vi "Process-images.vi"(8 "error in":errorcluster, 10 "UI ref. in":refnum<data-value>, 11 "Data ref. in":refnum<data-value>) -> (0 "error IO":errorcluster, 2 "UI ref.":refnum<data-value>, 3 "Data ref.":refnum<data-value>)   [LabVIEW 2013, in "CameraVision.lvlib" / "CV-Main.lvclass"]
uses:
  CV-Main.lvclass
  UI/CV-UI.lvclass
  UI/Module-states.ctl
  Buffers/Storage-buffer.ctl
  <vilib>/vision/Image Controls.llb/IMAQ Image.ctl
  Temperature/Temperature-characteristics.ctl
  Analysis/Characteristics-cluster.ctl
  Acquisition/Acquisition-stats.ctl
  UI/CV-UI.lvclass/CV-UI.ctl
  CV-Main.lvclass/CV-Main.ctl
  UI/Read Acquisition.vi
  Read Processing.vi
  Read UI buffer.vi
  Read Acq stats.vi
  Read Buffers.vi
  Read Config params.vi
  Read Correct params.vi
  Read Analysis params.vi
  Read Temperature params.vi
  Buffers/CV-Buffers.lvclass
  Configuration/CV-Configuration.lvclass
  Correction/CV-Correction.lvclass
  Analysis/CV-Analysis.lvclass
  Temperature/CV-Temperature.lvclass
  Acquisition/CV-Acquisition.lvclass
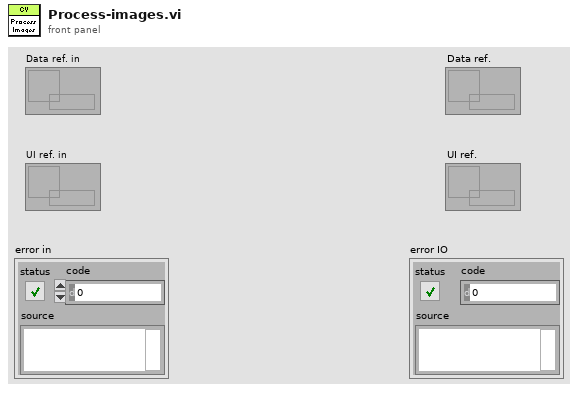
[diagram p1: front panel]
types:
  T1 = typedef "CameraVision.lvlib/CV-Acquisition.lvclass/Acquisition-stats.ctl" = cluster{"Index":i32, "Time":timestamp, "Acq duration":dbl, "Process duration":dbl}
  T2 = typedef "CameraVision.lvlib/CV-Buffers.lvclass/Storage-buffer.ctl" = cluster{"Index":i32, "Time":timestamp, "Raw images":T3[], "Corrected images":T3[], "Binary images":T3[], "Temperature characteristics":T4, "Characteristics":T5[], "Temperature field":dbl[][]}
  T3 = typedef "IMAQ Image.ctl" = refnum<image>
  T4 = typedef "CameraVision.lvlib/CV-Temperature.lvclass/Temperature-characteristics.ctl" = cluster{"Average temperature ":dbl, "Max. temperature":dbl, "Min. temperature":dbl, "Stand. dev. temperature":dbl, "Datapoints":dbl}
  T5 = typedef "CameraVision.lvlib/CV-Analysis.lvclass/Characteristics-cluster.ctl" = cluster{"Average intensity":dbl, "Peak intensity":dbl, "Melt-pool size":dbl, "Melt-pool aspect ratio":dbl, "Melt-pool fragments":dbl, "Centre of mass X":dbl, "Centre of mass Y":dbl, "Orientation":dbl}
  T6 = typedef "CameraVision.lvlib/CV-UI.lvclass/Module-states.ctl" = enum16{"Inactive", "Active", "Data-loss", "Error", "Simulation", "Synchronizing", "Initialized", "Released"}
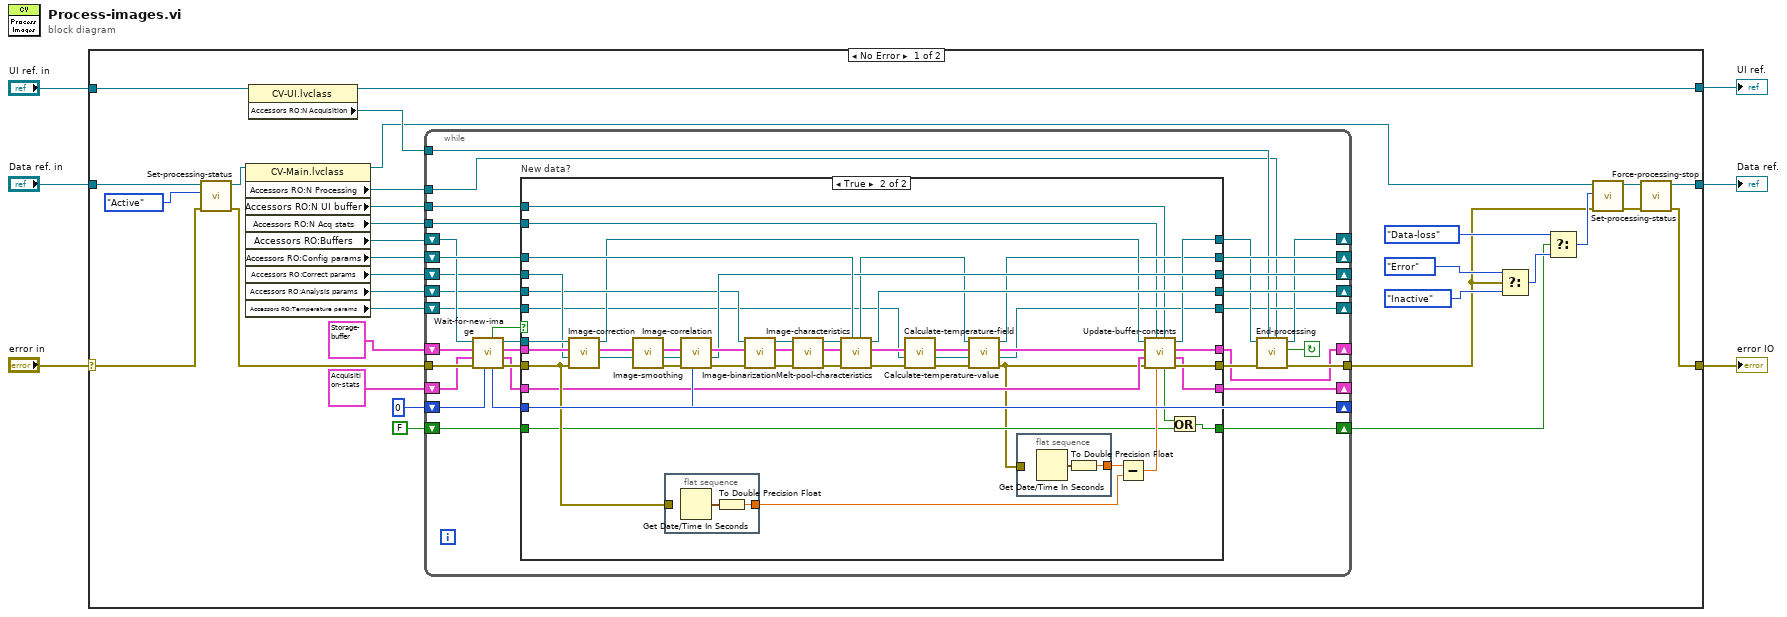
[diagram p0: block diagram]
diagram:
  n1 = case shown="No Error" "error in" {
    selector: "error in" -> [w25 w133]
    tunnel: [w10 w133] -> w6
    tunnel: "Data ref. in" -> [w35 w132]
    tunnel: "UI ref. in" -> [w34 w131]
    tunnel: [w33 w131] -> w2
    tunnel: [w9 w132] -> w1
    frame No Error {
      n2 = call "Set-processing-status.vi"("error in"=w25, "Process. status in"=Module-states."Active" ("Basic proc. status"), "Data ref. in"=w35) -> ("error IO"=w18:errorcluster, "Data ref."=w26:refnum<data-value>)  [unwired: 6 in, 1 out]
      n3 = property class="CV-Main.lvclass"(reference=w26) -> (reference out=w32:refnum<data-value>, "Accessors RO:N Processing"=w7:refnum<notifier>, "Accessors RO:N UI buffer"=w8:refnum<notifier>, "Accessors RO:N Acq stats"=w14:refnum<notifier>, "Accessors RO:Buffers"=w31:refnum<class "CV-Buffers.lvclass">, "Accessors RO:Config params"=w30:refnum<data-value>, "Accessors RO:Correct params"=w29:refnum<data-value>, "Accessors RO:Analysis params"=w28:refnum<data-value>, "Accessors RO:Temperature params"=w15:refnum<data-value>)  [unwired: 1 in, 1 out]
      n4 = property class="CV-UI.lvclass"(reference=w34) -> (reference out=w33:refnum<data-value>, "Accessors RO:N Acquisition"=w36:refnum<notifier>)  [unwired: 1 in, 1 out]
      n5 = while {
        tunnel: w18 -> [w68]
        tunnel: [w70] -> w13
        shift-right: [w45] -> _
        shift-left: w31 -> [w64]
        shift-right: [w66] -> _
        shift-left: w30 -> [w69]
        shift-right: [w58] -> _
        shift-left: w29 -> [w60]
        shift-right: [w53] -> _
        shift-left: w28 -> [w57]
        shift-right: [w55] -> _
        shift-left: 0 -> [w65]
        shift-right: [w47] -> w20
        shift-left: FALSE -> [w48]
        shift-right: [w49] -> _
        shift-left: T2 {"Index"=0, "Time"=timestamp(0 s since 1904-01-01), "Raw images"=[], "Corrected images"=[], "Binary images"=[], "Temperature characteristics"={"Average temperature "=0.0, "Max. temperature"=0.0, "Min. temperature"=0.0, "Stand. dev. temperature"=0.0, "Datapoints"=0.0}, "Characteristics"=[], "Temperature field"=[]} ("Storage element") -> [w59]
        shift-right: [w51] -> _
        shift-left: T1 {"Index"=0, "Time"=timestamp(0 s since 1904-01-01), "Acq duration"=0.0, "Process duration"=0.0} ("Acq. stats in") -> [w56]
        tunnel: w14 -> [w54]
        tunnel: w36 -> [w46]
        shift-right: [w42] -> _
        shift-left: w15 -> [w43]
        tunnel: w8 -> [w41]
        tunnel: w7 -> [w39]
        stop <- w40 continue-if-true
        n6 = call "Wait-for-new-image.vi"("Index in"=w65, "error in"=w68, "Acq. stats in"=w56, "Buffer element in"=w59, "Buffers in"=w64) -> ("error IO"=w62:errorcluster, "Acq. stats"=w52:T1, "Buffer element"=w63:T2, "Buffers"=w61:refnum<class "CV-Buffers.lvclass">, "Index"=w55:i32, "New data?"=w50:bool)  [unwired: 1 in]
        n7 = case "New data?" shown="True" w50 {
          tunnel: w69 -> [w79 w126]
          tunnel: [w74 w125] -> w67
          tunnel: [w79 w84] -> w66
          tunnel: w63 -> [w73 w122]
          tunnel: w62 -> [w74 w121]
          tunnel: w61 -> [w76 w120]
          tunnel: w60 -> [w78 w119]
          tunnel: [w78 w105] -> w58
          tunnel: w57 -> [w77 w104]
          tunnel: w55 -> [_ w103]
          tunnel: [w76 w96] -> w44
          tunnel: w54 -> [_ w80]
          tunnel: [w77 w101] -> w53
          tunnel: w52 -> [w75 w100]
          tunnel: [w75 w99] -> w51
          tunnel: [w73 w98] -> w49
          tunnel: w48 -> [w72 w95]
          tunnel: [w72 w94] -> w47
          tunnel: w43 -> [w71 w83]
          tunnel: [w71 w82] -> w42
          tunnel: w41 -> [_ w81]
          frame False {
          }
          frame True {
            n8 = call "Image-correction.vi"("error in"=w121, "Correct. params. ref. in"=w119, "Buffer element in"=w122, "Buffers in"=w120) -> ("Correct. params. ref."=w114:refnum<data-value>, "Buffer element"=w115:T2, "Buffers"=w97:refnum<class "CV-Buffers.lvclass">)  [unwired: 4 in, 1 out]
            n9 = call "Image-smoothing.vi"("Correct. params. ref. in"=w114, "Buffer element in"=w115) -> ("error IO"=w118:errorcluster, "Correct. params. ref."=w117:refnum<data-value>, "Buffer element"=w116:T2)  [unwired: 7 in]
            n10 = flat-sequence {
              tunnel: w121 -> [_]
              tunnel: [w129] -> w124
              frame #0 {
                n11 = Get Date/Time In Seconds() -> (seconds since 1Jan1904=w130:timestamp)
                n12 = To Double Precision Float(number=w130) -> (double precision float=w129:dbl)
              }
            }
            n13 = call "Image-correlation.vi"("Image index"=w103, "error in"=w118, "Correct. params. ref. in"=w117, "Buffer element in"=w116) -> ("error IO"=w112:errorcluster, "Correct. params. ref."=w105:refnum<data-value>, "Buffer element"=w113:T2)  [unwired: 5 in]
            n14 = call "Image-binarization.vi"("error in"=w112, "Buffer element in"=w113, "Analysis params. ref. in"=w104) -> ("error IO"=w111:errorcluster, "Buffer element"=w110:T2, "Analysis params. ref."=w109:refnum<data-value>)  [unwired: 6 in]
            n15 = call "Image-characteristics.vi"("error in"=w111, "Buffer element in"=w110, "Analysis params. ref. in"=w109) -> ("error IO"=w106:errorcluster, "Buffer element"=w107:T2, "Analysis params. ref."=w108:refnum<data-value>)  [unwired: 6 in]
            n16 = call "Melt-pool-characteristics.vi"("Config. params. ref. in"=w126, "error in"=w106, "Buffer element in"=w107, "Analysis params. ref. in"=w108) -> ("error IO"=w91:errorcluster, "Buffer element"=w92:T2, "Analysis params. ref."=w101:refnum<data-value>, "Config. params. ref."=w85:refnum<data-value>)  [unwired: 4 in]
            n17 = call "Calculate-temperature-field.vi"("error in"=w91, "Temp. params. ref. in"=w83, "Buffer element in"=w92) -> ("error IO"=w86:errorcluster, "Temp. params. ref."=w90:refnum<data-value>, "Buffer element"=w89:T2)  [unwired: 6 in]
            n18 = call "Calculate-temperature-value.vi"("error in"=w86, "Temp. params. ref. in"=w90, "Buffer element in"=w89, "Config. params. ref. in"=w85) -> ("error IO"=w87:errorcluster, "Temp. params. ref."=w82:refnum<data-value>, "Buffer element"=w88:T2, "Config. params. ref."=w84:refnum<data-value>)  [unwired: 4 in]
            n19 = flat-sequence {
              tunnel: [w127] -> w123
              tunnel: w87 -> [_]
              frame #0 {
                n20 = Get Date/Time In Seconds() -> (seconds since 1Jan1904=w128:timestamp)
                n21 = To Double Precision Float(number=w128) -> (double precision float=w127:dbl)
              }
            }
            n22 = Subtract(x=w123, y=w124) -> (x-y=w102:dbl)
            n23 = call "Update-buffer-contents.vi"("UI buffer"=w81, "Frametime"=w102, "Acq stats notif"=w80, "error in"=w87, "Acquisition stats in"=w100, "Buffer element in"=w88, "Buffers in"=w97) -> ("error IO"=w125:errorcluster, "Acquisition stats"=w99:T1, "Buffer element"=w98:T2, "Buffers"=w96:refnum<class "CV-Buffers.lvclass">, "Data-loss?"=w93:bool)
            n24 = Or(x=w93, y=w95) -> (x .or. y?=w94:bool)
          }
        }
        n25 = call "End-processing.vi"("Processing?"=w39, "Acquiring?"=w46, "error in"=w67, "Buffers in"=w44) -> ("error IO"=w70:errorcluster, "Continue processing?"=w40:bool, "Buffers"=w45:refnum<class "CV-Buffers.lvclass">)  [unwired: 5 in]
      }
      n26 = Select(t=Module-states."Error" ("Basic proc. status"), s=w13, f=Module-states."Inactive" ("Basic proc. status")) -> (s? t:f=w22:T6)
      n27 = Select(t=Module-states."Data-loss" ("Basic proc. status"), s=w20, f=w22) -> (s? t:f=w19:T6)
      n28 = call "Set-processing-status.vi"("error in"=w13, "Process. status in"=w19, "Data ref. in"=w32) -> ("error IO"=w11:errorcluster, "Data ref."=w12:refnum<data-value>)  [unwired: 6 in, 1 out]
      n29 = call "Force-processing-stop.vi"("error in"=w11, "Data ref. in"=w12) -> ("error IO"=w10:errorcluster, "Data ref."=w9:refnum<data-value>)  [unwired: 8 in]
    }
    frame Error {
    }
  }
  "error IO" <- w6
  "Data ref." <- w1
  "UI ref." <- w2
